vi "UI.vi"() -> ()   [LabVIEW 2017]
uses:
  <vilib>/vision/NI_Vision_Development_Module.lvlib
panel:
  out "D_damaged 4":ext
  out "D_giltch 4":ext
  out "D_damaged 3":ext
  out "D_giltch 3":ext
  out "D_damaged 2":ext
  out "D_giltch 2":ext
  out "D_damaged":ext
  out "D_giltch":ext
  in  "side length (mm)":dbl
  in  "Path":path
  in  "Main Range (Threshold)":cluster{"Lower value":sgl, "Upper value":sgl}={"Lower value"=73.0, "Upper value"=255.0}
  out "display image":T1(plugin-control)
  in  "image imshow":bool
  out "time image processing":u32
  out "time load image":u32
  out "Y Resolution":i32
  out "X Resolution":i32
  out "black image":T1(plugin-control)
  out "buffer image":T1(plugin-control)
  in  "Sub Range (Threshold)":cluster{"Lower value":sgl, "Upper value":sgl}={"Lower value"=73.0, "Upper value"=255.0}
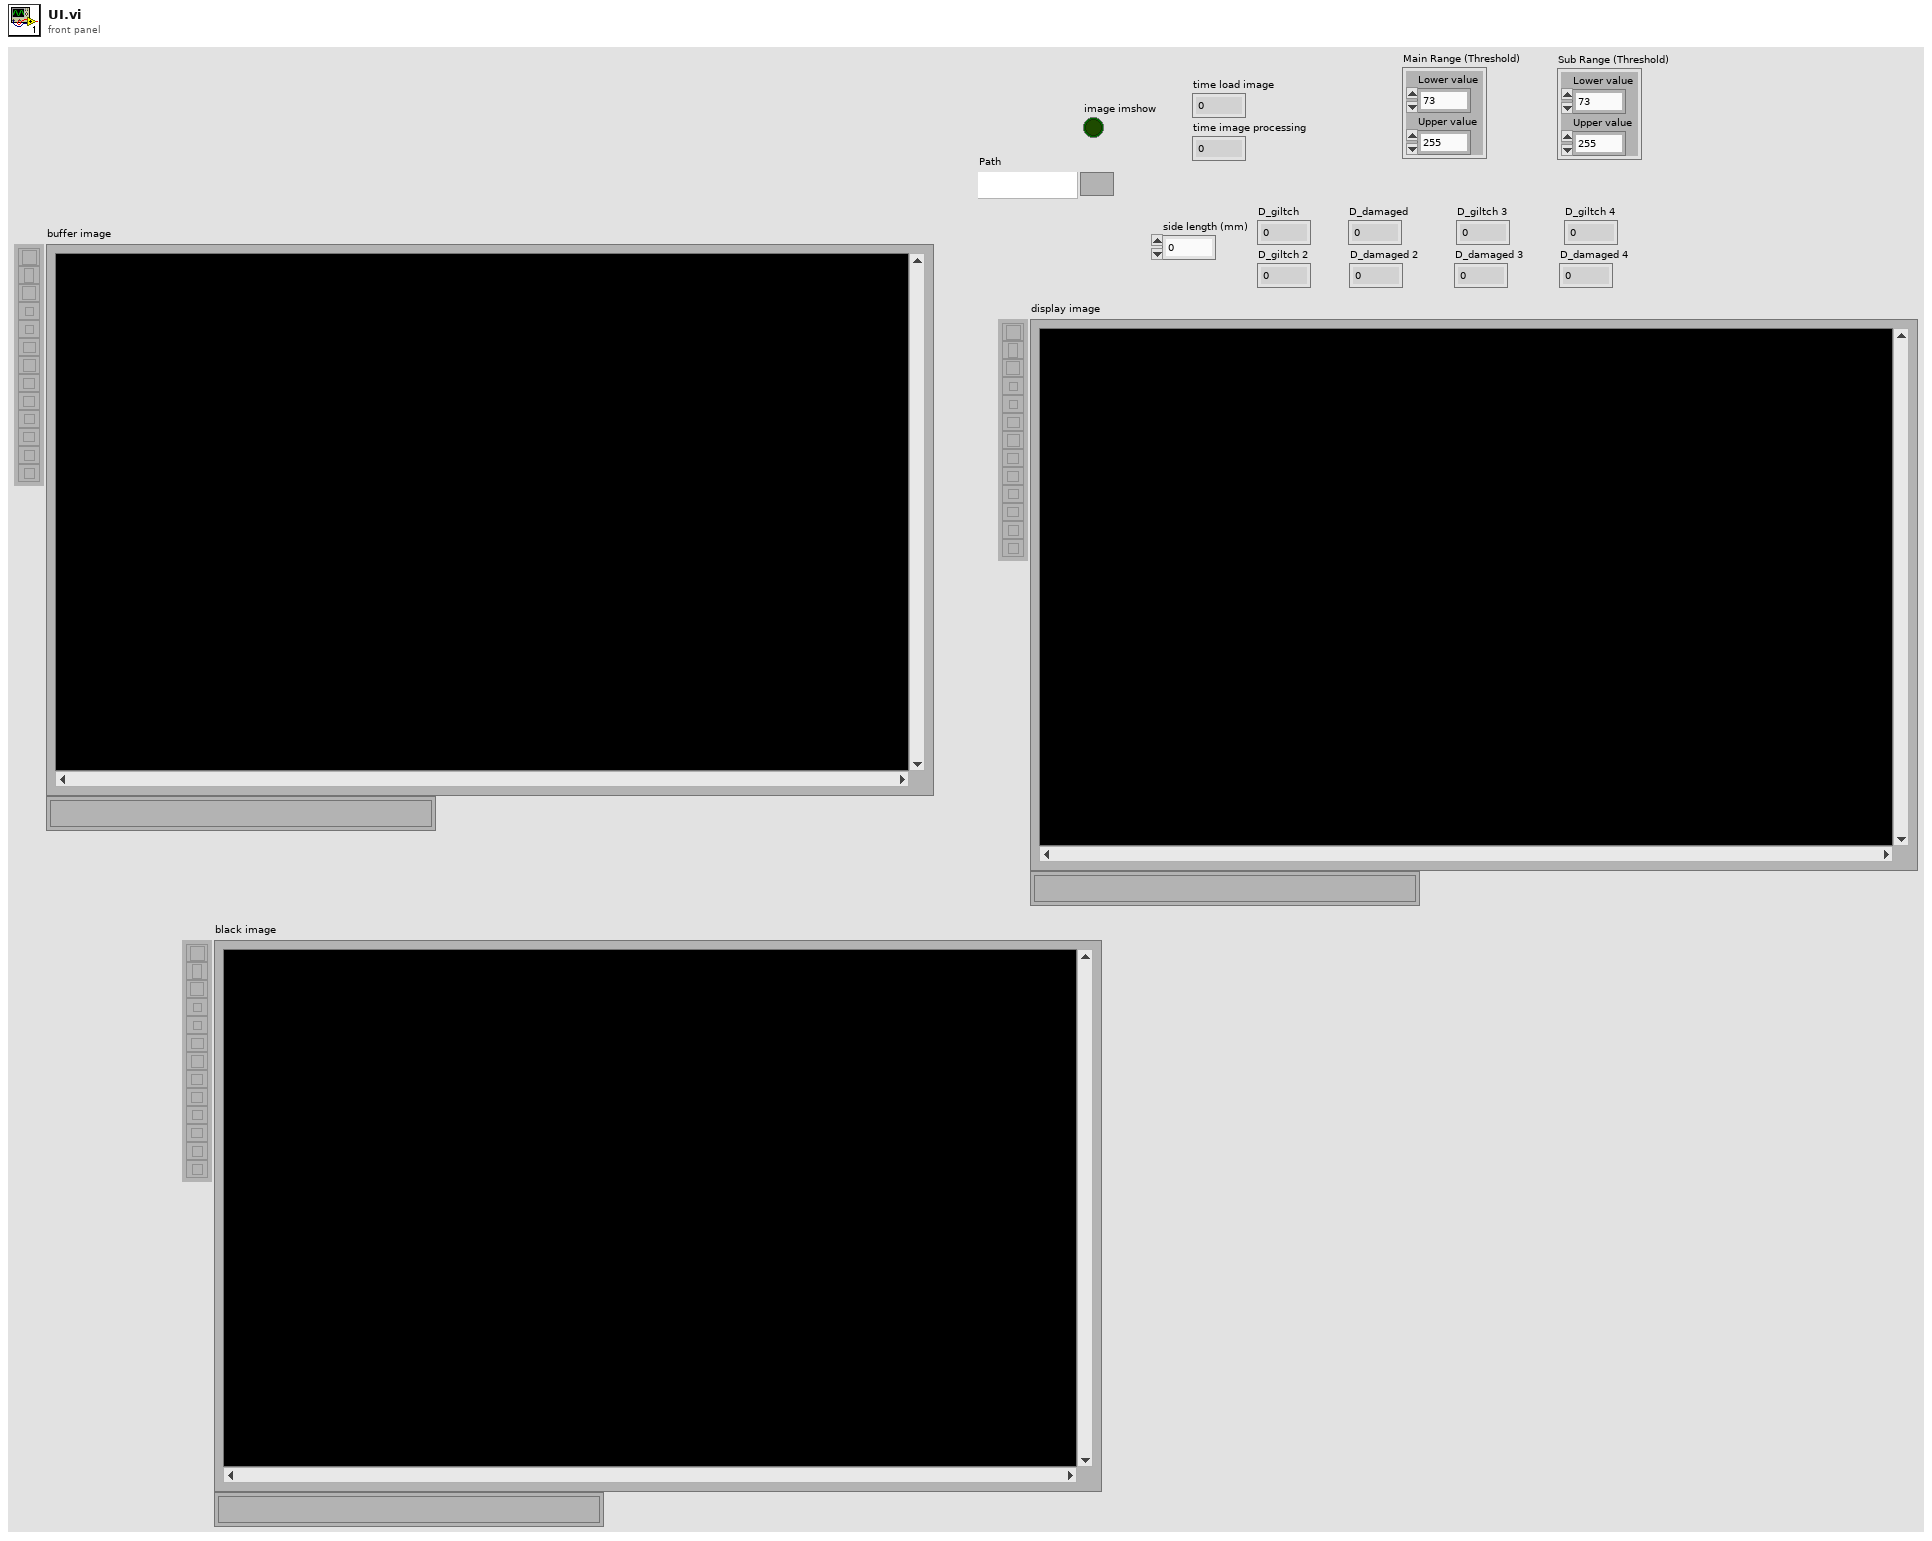
[diagram p1: front panel]
types:
  T1 = typedef "IMAQ Image.ctl" = refnum<image>
  T2 = enum32{"AutoM", "Close", "Dilate", "Erode", "Gradient", "Gradient out", "Gradient in", "Hit miss", "Open", "PClose", "POpen", "Thick", "Thin"}
  T3 = cluster{"Sigma":sgl, "HThresh":sgl, "LThres":sgl, "WindowSize":i32}
  T4 = cluster{"Number of Points":i32, "Open/Closed":i32, "Weight":dbl, "Contour Points":cluster{"X":dbl, "Y":dbl, "Curvature":dbl, "X Displacement":dbl, "Y Displacement":dbl}[]}[]
  T5 = cluster{"Left":i32, "Top":i32, "Right":i32, "Bottom":i32}
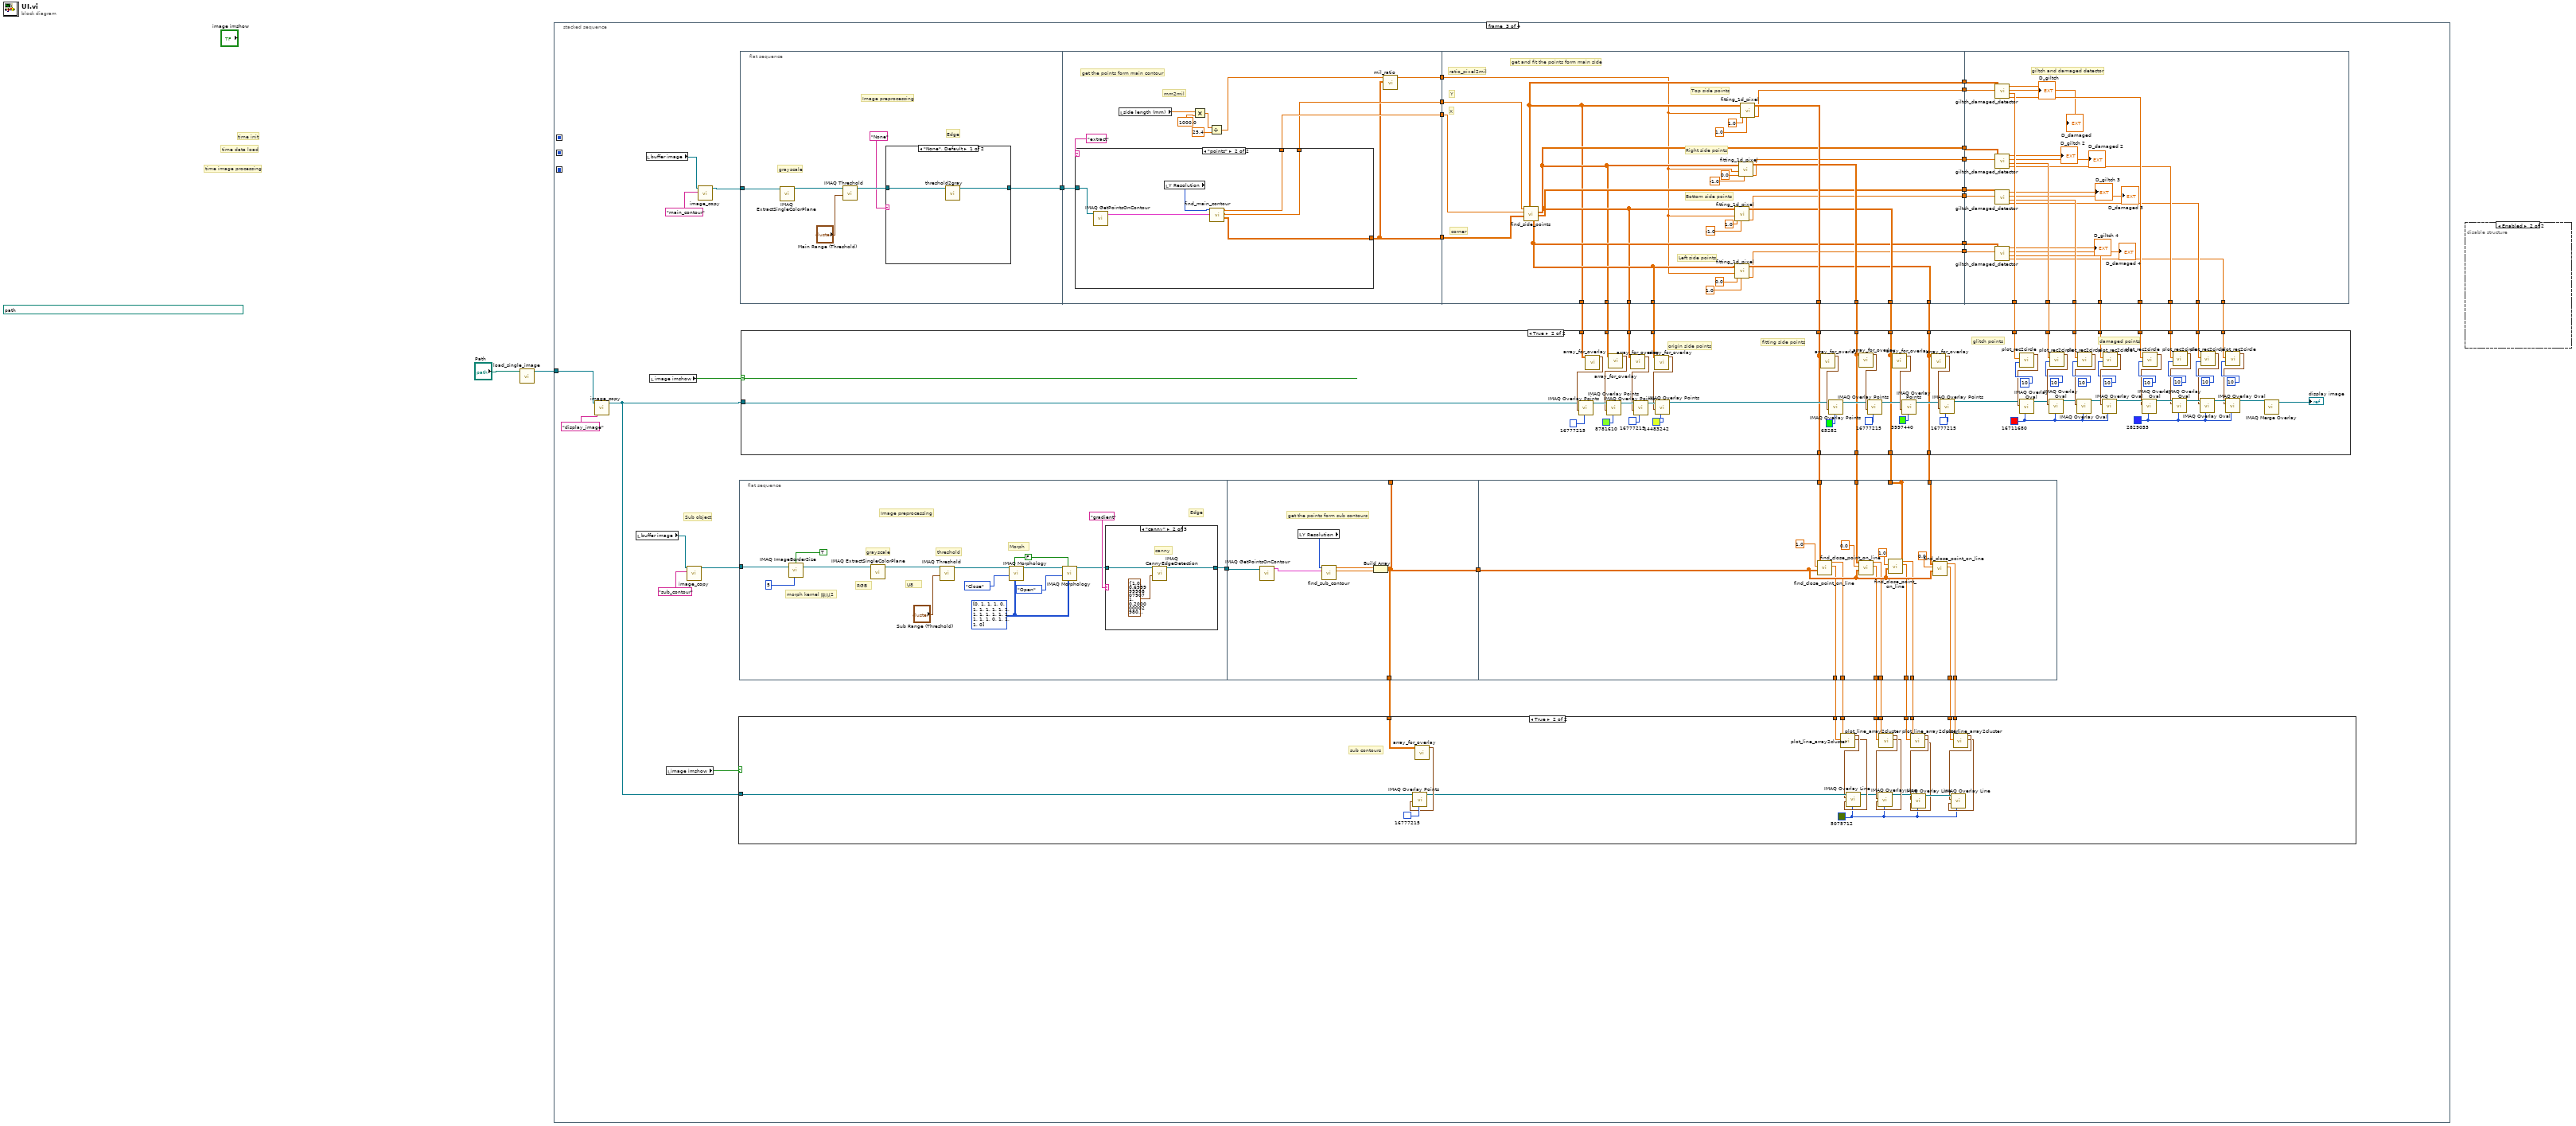
[diagram p0: block diagram]
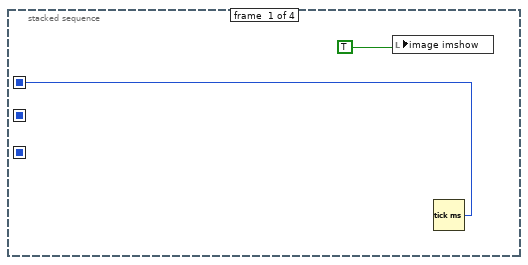
[diagram p2: hidden frame]
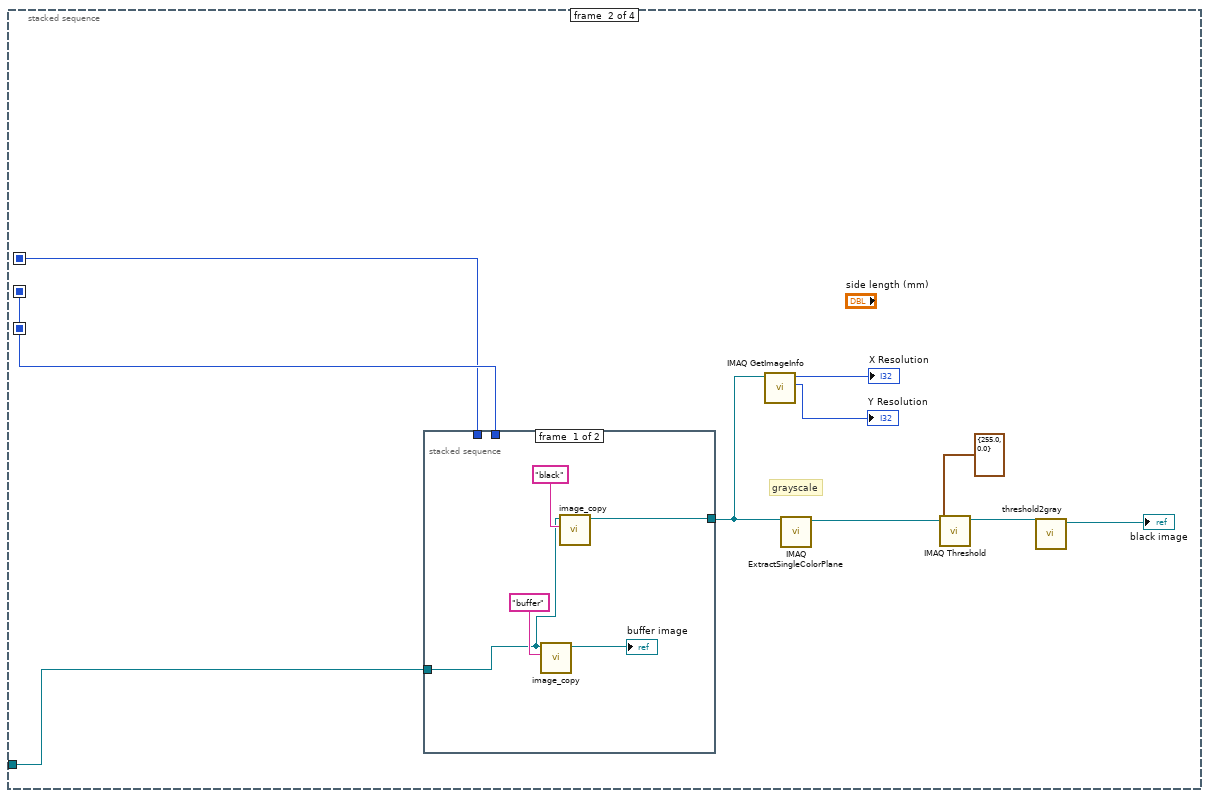
[diagram p3: hidden frame]
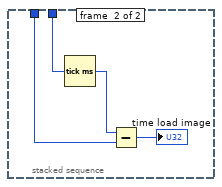
[diagram p4: hidden frame]
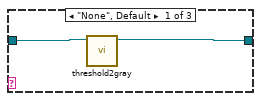
[diagram p6: hidden frame]
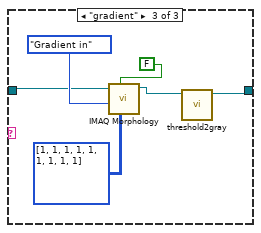
[diagram p7: hidden frame]
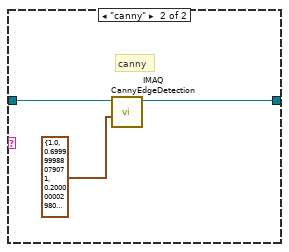
[diagram p8: hidden frame]
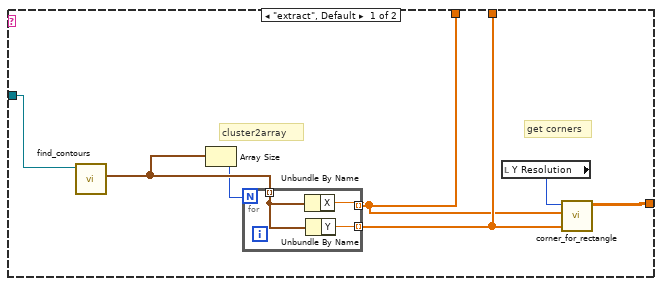
[diagram p9: hidden frame]
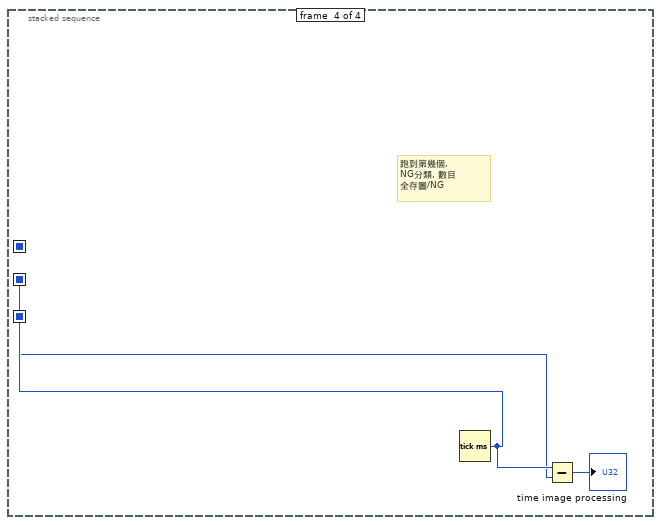
[diagram p11: hidden frame]
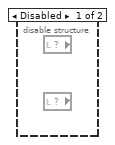
[diagram p12: hidden frame]
diagram:
  (unwired) path "X:/liteon_repeater/labview/G163良品及不良照片/labview_code/test_img/bottom-damage-1.png" ("Path")
  # "time image processing"
  # "time data load"
  # "time init"
  n1 = call "load_single_image.vi"("Path"="Path") -> ("Refnum out"=w2:T1)  [unwired: 10 in]
  n2 = stacked-sequence {
    seq-local: [w4 _ _ _] -> [_ w7 _ _]
    seq-local: [_ w8 _ _] -> [_ _ _ w311]
    seq-local: [_ _ _ w312] -> [_ _ _ _]
    tunnel: w2 -> [_ w9 w34 _]
    frame #0 {
      n3 = local write "image imshow"(TRUE) -> ()
      n4 = Tick Count (ms)() -> (millisecond timer value=w4:u32)
    }
    frame #1 {
      # "grayscale"
      n5 = stacked-sequence {
        tunnel: [w17 _] -> w12
        tunnel: w9 -> [w16 _]
        tunnel: [_ w22] -> w8
        tunnel: w7 -> [_ w21]
        frame #0 {
          n6 = call "image_copy.vi"("buffer name"="buffer" ("Image Name"), "image in"=w16) -> ("imgae out"=→"buffer image":T1)  [unwired: 9 in]
          n7 = call "image_copy.vi"("buffer name"="black" ("Image Name"), "image in"=w16) -> ("imgae out"=w17:T1)  [unwired: 9 in]
        }
        frame #1 {
          n8 = Tick Count (ms)() -> (millisecond timer value=w22:u32)
          n9 = Subtract(x=w22, y=w21) -> (x-y=→"time load image":u32)
        }
      }
      n10 = call "IMAQ GetImageInfo"("Image"=w12) -> ("Y Resolution"=→"Y Resolution":i32, "X Resolution"=→"X Resolution":i32)  [unwired: 3 in, 6 out]
      n11 = call "IMAQ ExtractSingleColorPlane"("Image Src"=w12) -> ("Image Dst Out"=w14:T1)  [unwired: 3 in, 7 out]
      n12 = call "IMAQ Threshold"("Range"=cluster{"Lower value":sgl, "Upper value":sgl} {"Lower value"=255.0, "Upper value"=0.0}, "Image Src"=w14) -> ("Image Dst Out"=w6:T1)  [unwired: 4 in, 5 out]
      n13 = call "threshold2gray.vi"("threshold image"=w6) -> ("grayscale image"=→"black image":T1)  [unwired: 10 in]
    }
    frame #2 {
      # "Sub object"
      n14 = call "image_copy.vi"("buffer name"="display_image" ("Image Name"), "image in"=w34) -> ("imgae out"=w33:T1)  [unwired: 9 in]
      n15 = local read "buffer image"() -> (w64:T1)
      n16 = local read "buffer image"() -> (w75:T1)
      n17 = local read "image imshow"() -> (w77:bool)
      n18 = local read "image imshow"() -> (w30:bool)
      n19 = call "image_copy.vi"("buffer name"="sub_contour" ("Image Name"), "image in"=w64) -> ("imgae out"=w63:T1)  [unwired: 9 in]
      n20 = call "image_copy.vi"("buffer name"="main_contour" ("Image Name"), "image in"=w75) -> ("imgae out"=w74:T1)  [unwired: 9 in]
      n21 = case shown="True" w30 {
        tunnel: w33 -> [_ w100]
        tunnel: w32 -> [_ w99]
        tunnel: w31 -> [_ w98]
        tunnel: w29 -> [_ w96]
        tunnel: w28 -> [_ w94]
        tunnel: w27 -> [_ w92]
        tunnel: w26 -> [_ w97]
        tunnel: w25 -> [_ w95]
        tunnel: w24 -> [_ w93]
        tunnel: w23 -> [_ w91]
        frame False {
        }
        frame True {
          w78 = u32 5075712 ("Color")
          # "sub contours"
          n22 = call "array_for_overlay.vi"("Array in"=w99) -> ("Array out"=w101:cluster{"X":i32, "Y":i32}[])  [unwired: 10 in]
          n23 = call "IMAQ Overlay Points"("Color"=u32 16777215, "Array of Points"=w101, "Image"=w100) -> ("Image Out"=w90:T1)  [unwired: 7 in, 1 out]
          n24 = call "plot_line_array2cluster.vi"("End Point array"=w98, "Start Point array"=w97) -> ("End Point out"=w88:cluster{"X":i32, "Y":i32}, "Start Point out"=w89:cluster{"X":i32, "Y":i32})  [unwired: 8 in]
          n25 = call "IMAQ Overlay Line"("Color"=w78, "End Point"=w88, "Start Point"=w89, "Image"=w90) -> ("Image Out"=w85:T1)  [unwired: 6 in, 1 out]
          n26 = call "plot_line_array2cluster.vi"("End Point array"=w96, "Start Point array"=w95) -> ("End Point out"=w86:cluster{"X":i32, "Y":i32}, "Start Point out"=w87:cluster{"X":i32, "Y":i32})  [unwired: 8 in]
          n27 = call "IMAQ Overlay Line"("Color"=w78, "End Point"=w86, "Start Point"=w87, "Image"=w85) -> ("Image Out"=w84:T1)  [unwired: 6 in, 1 out]
          n28 = call "plot_line_array2cluster.vi"("End Point array"=w94, "Start Point array"=w93) -> ("End Point out"=w81:cluster{"X":i32, "Y":i32}, "Start Point out"=w82:cluster{"X":i32, "Y":i32})  [unwired: 8 in]
          n29 = call "IMAQ Overlay Line"("Color"=w78, "End Point"=w81, "Start Point"=w82, "Image"=w84) -> ("Image Out"=w83:T1)  [unwired: 6 in, 1 out]
          n30 = call "plot_line_array2cluster.vi"("End Point array"=w92, "Start Point array"=w91) -> ("End Point out"=w79:cluster{"X":i32, "Y":i32}, "Start Point out"=w80:cluster{"X":i32, "Y":i32})  [unwired: 8 in]
          n31 = call "IMAQ Overlay Line"("Color"=w78, "End Point"=w79, "Start Point"=w80, "Image"=w83) -> ()  [unwired: 6 in, 2 out]
        }
      }
      n32 = flat-sequence {
        tunnel: w63 -> [w112]
        tunnel: [w108] -> w62
        tunnel: w62 -> [w134]
        tunnel: [w129] -> _
        tunnel: [w129] -> w36
        tunnel: [w129] -> w32
        tunnel: w40 -> [w145]
        tunnel: w39 -> [w149]
        tunnel: [w148] -> _
        tunnel: w38 -> [w148]
        tunnel: w37 -> [w146]
        tunnel: w36 -> [w147]
        tunnel: [w142] -> w31
        tunnel: [w141] -> w29
        tunnel: [w140] -> w28
        tunnel: [w139] -> w27
        tunnel: [w138] -> w26
        tunnel: [w137] -> w25
        tunnel: [w136] -> w24
        tunnel: [w135] -> w23
        frame #0 {
          w105 = i32[][] [[0, 1, 1, 1, 0], [1, 1, 1, 1, 1], [1, 1, 1, 1, 1], [1, 1, 1, 1, 1], [0, 1, 1, 1, 0]] ("Structuring Element")
          w106 = FALSE ("Square/Hexa (Square)")
          # "Image preprocessing"
          # "Morph"
          # "morph kernel 除以2"
          # "Edge"
          # "U8"
          # "RGB"
          # "threshold"
          # "grayscale"
          n33 = call "IMAQ ImageBorderSize"("Get/Set Status? (Set)"=TRUE, "Image"=w112, "Image border size in"=5) -> ("Image Out"=w111:T1)  [unwired: 1 in, 2 out]
          n34 = call "IMAQ ExtractSingleColorPlane"("Image Src"=w111) -> ("Image Dst Out"=w116:T1)  [unwired: 3 in, 7 out]
          n35 = call "IMAQ Threshold"("Range"="Sub Range (Threshold)", "Image Src"=w116) -> ("Image Dst Out"=w113:T1)  [unwired: 4 in, 5 out]
          n36 = call "IMAQ Morphology"("Structuring Element"=w105, "Square/Hexa (Square)"=w106, "Operation"=T2."Close", "Image Src"=w113) -> ("Image Dst Out"=w103:T1)  [unwired: 3 in, 4 out]
          n37 = call "IMAQ Morphology"("Structuring Element"=w105, "Square/Hexa (Square)"=w106, "Operation"=T2."Open", "Image Src"=w103) -> ("Image Dst Out"=w104:T1)  [unwired: 3 in, 4 out]
          n38 = case shown="\"canny\"" "gradient" {
            tunnel: [w118 w122 w123] -> w108
            tunnel: w104 -> [w119 w121 w125]
            frame "None", Default {
              n39 = call "threshold2gray.vi"("threshold image"=w119) -> ("grayscale image"=w118:T1)  [unwired: 10 in]
            }
            frame "canny" {
              # "canny"
              n40 = call "IMAQ CannyEdgeDetection"("Image Src"=w121, "Filter Parameters"=T3 {"Sigma"=1.0, "HThresh"=0.7, "LThres"=0.2, "WindowSize"=9}) -> ("Image Dst Out"=w122:T1)  [unwired: 2 in, 5 out]
            }
            frame "gradient" {
              n41 = call "IMAQ Morphology"("Structuring Element"=i32[][] [[1, 1, 1], [1, 1, 1], [1, 1, 1]], "Square/Hexa (Square)"=FALSE, "Operation"=T2."Gradient in", "Image Src"=w125) -> ("Image Dst Out"=w124:T1)  [unwired: 3 in, 4 out]
              n42 = call "threshold2gray.vi"("threshold image"=w124) -> ("grayscale image"=w123:T1)  [unwired: 10 in]
            }
          }
        }
        frame #1 {
          # "get the points form sub contours"
          n43 = call "IMAQ GetPointsOnContour"("Image (Edge Image)"=w134) -> ("Segment Information"=w133:T4)  [unwired: 3 in, 2 out]
          n44 = local read "Y Resolution"() -> (w132:i32)
          n45 = call "find_sub_contour.vi"("Segment Information"=w133, "Y Resolution"=w132) -> ("Y"=w130:dbl[], "X"=w131:dbl[])  [unwired: 8 in]
          n46 = Build Array(w131, w130) -> (w129:dbl[][])
        }
        frame #2 {
          n47 = call "find_close_point_on_line.vi"("Array in"=w147, "fitting axis"=1.0, "fitting array"=w145) -> ("XY online"=w142:dbl[], "XY point"=w138:dbl[])  [unwired: 6 in, 1 out]
          n48 = call "find_close_point_on_line.vi"("Array in"=w147, "fitting axis"=0.0, "fitting array"=w149) -> ("XY online"=w141:dbl[], "XY point"=w137:dbl[])  [unwired: 6 in, 1 out]
          n49 = call "find_close_point_on_line.vi"("Array in"=w147, "fitting axis"=1.0, "fitting array"=w148) -> ("XY online"=w140:dbl[], "XY point"=w136:dbl[])  [unwired: 6 in, 1 out]
          n50 = call "find_close_point_on_line.vi"("Array in"=w147, "fitting axis"=0.0, "fitting array"=w146) -> ("XY online"=w139:dbl[], "XY point"=w135:dbl[])  [unwired: 6 in, 1 out]
        }
      }
      n51 = flat-sequence {
        tunnel: w74 -> [w156]
        tunnel: [w153] -> w73
        tunnel: w73 -> [w172]
        tunnel: [w165] -> w72
        tunnel: [w171] -> w67
        tunnel: [w170] -> w66
        tunnel: [w163] -> w41
        tunnel: w72 -> [w213]
        tunnel: [w191] -> w71
        tunnel: [w193] -> w70
        tunnel: [w195] -> w69
        tunnel: [w197] -> w68
        tunnel: w67 -> [w212]
        tunnel: w66 -> [w211]
        tunnel: [w209] -> w61
        tunnel: [w205] -> w60
        tunnel: [w204] -> w59
        tunnel: [w203] -> w58
        tunnel: [w198] -> w57
        tunnel: [w197] -> w56
        tunnel: [w196] -> w55
        tunnel: [w195] -> w54
        tunnel: [w194] -> w53
        tunnel: [w193] -> w52
        tunnel: [w192] -> w51
        tunnel: [w191] -> w50
        tunnel: w41 -> [w190]
        tunnel: w57 -> [w237]
        tunnel: w56 -> [w236]
        tunnel: w55 -> [w235]
        tunnel: w54 -> [w234]
        tunnel: w53 -> [w233]
        tunnel: w52 -> [w232]
        tunnel: w51 -> [w231]
        tunnel: w50 -> [w230]
        tunnel: [w229] -> w49
        tunnel: [w228] -> w48
        tunnel: [w227] -> w47
        tunnel: [w226] -> w46
        tunnel: [w225] -> w45
        tunnel: [w224] -> w44
        tunnel: [w223] -> w43
        tunnel: [w222] -> w42
        frame #0 {
          # "Image preprocessing"
          # "grayscale"
          # "Edge"
          n52 = call "IMAQ ExtractSingleColorPlane"("Image Src"=w156) -> ("Image Dst Out"=w155:T1)  [unwired: 3 in, 7 out]
          n53 = call "IMAQ Threshold"("Range"="Main Range (Threshold)", "Image Src"=w155) -> ("Image Dst Out"=w154:T1)  [unwired: 4 in, 5 out]
          n54 = case shown="\"None\", Default" "None" {
            tunnel: [w158 w162] -> w153
            tunnel: w154 -> [w159 w161]
            frame "None", Default {
              n55 = call "threshold2gray.vi"("threshold image"=w159) -> ("grayscale image"=w158:T1)  [unwired: 10 in]
            }
            frame "canny" {
              # "canny"
              n56 = call "IMAQ CannyEdgeDetection"("Image Src"=w161, "Filter Parameters"=T3 {"Sigma"=1.0, "HThresh"=0.7, "LThres"=0.2, "WindowSize"=9}) -> ("Image Dst Out"=w162:T1)  [unwired: 2 in, 5 out]
            }
          }
        }
        frame #1 {
          # "mm2mil"
          # "get the points form main contour"
          n57 = case shown="\"points\"" "extract" {
            tunnel: w172 -> [w176 w189]
            tunnel: [w177 w184] -> w165
            tunnel: [w175 w185] -> w170
            tunnel: [w174 w186] -> w171
            frame "extract", Default {
              # "get corners"
              # "cluster2array"
              n58 = call "find_contours.vi"("image in"=w176) -> ("Source Image Points"=w180:cluster{"X":dbl, "Y":dbl}[])  [unwired: 9 in, 1 out]
              n59 = Array Size(array=w180) -> (size(s)=w178:i32)
              n60 = for {
                N: w178 -> [_]
                tunnel: w180 -> [w182] mode=indexing
                tunnel: [w183] -> w174 mode=indexing
                tunnel: [w181] -> w175 mode=indexing
                n61 = Unbundle By Name(w182) -> ("X"=w183:dbl)
                n62 = Unbundle By Name(w182) -> ("Y"=w181:dbl)
              }
              n63 = local read "Y Resolution"() -> (w179:i32)
              n64 = call "corner_for_rectangle.vi"("Y"=w175, "X"=w174, "Y Resolution"=w179) -> ("corner"=w177:dbl[][])  [unwired: 7 in, 1 out]
            }
            frame "points" {
              n65 = call "IMAQ GetPointsOnContour"("Image (Edge Image)"=w189) -> ("Segment Information"=w187:T4)  [unwired: 3 in, 2 out]
              n66 = local read "Y Resolution"() -> (w188:i32)
              n67 = call "find_main_contour.vi"("Segment Information"=w187, "Y Resolution"=w188) -> ("max corner"=w184:dbl[][], "Y"=w185:dbl[], "X"=w186:dbl[])  [unwired: 7 in]
            }
          }
          n68 = local read "side length (mm)"() -> (w168:dbl)
          n69 = Multiply(x=w168, y=1000.0) -> (x*y=w167:dbl)
          n70 = Divide(x=w167, y=25.4) -> (x/y=w164:dbl)
          n71 = call "mil_ratio.vi"("corner"=w165, "mil"=w164) -> ("ratio"=w163:dbl)  [unwired: 9 in]
        }
        frame #2 {
          # "corner"
          # "X"
          # "Y"
          # "ratio_pixel2mil"
          # "Left side points"
          # "Bottom side points"
          # "Right side points"
          # "Top side points"
          # "get and fit the points form main side"
          n72 = call "find_side_points.vi"("corner"=w213, "X  coords array"=w212, "Y coords array"=w211) -> ("Bottom side points"=w195:dbl[][], "Right side points"=w193:dbl[][], "Top side points"=w191:dbl[][], "Left side points"=w197:dbl[][])  [unwired: 5 in]
          n73 = call "fitting_1d_pixel.vi"("D sign"=-1.0, "fitting axis"=1.0, "ratio_pixel2mil"=w190, "array in"=w195) -> ("D"=w196:ext[], "fitting array"=w204:dbl[][])  [unwired: 6 in]
          n74 = call "fitting_1d_pixel.vi"("D sign"=1.0, "fitting axis"=0.0, "ratio_pixel2mil"=w190, "array in"=w197) -> ("D"=w198:ext[], "fitting array"=w203:dbl[][])  [unwired: 6 in]
          n75 = call "fitting_1d_pixel.vi"("D sign"=-1.0, "fitting axis"=0.0, "ratio_pixel2mil"=w190, "array in"=w193) -> ("D"=w194:ext[], "fitting array"=w205:dbl[][])  [unwired: 6 in]
          n76 = call "fitting_1d_pixel.vi"("D sign"=1.0, "fitting axis"=1.0, "ratio_pixel2mil"=w190, "array in"=w191) -> ("D"=w192:ext[], "fitting array"=w209:dbl[][])  [unwired: 6 in]
        }
        frame #3 {
          # "giltch and damaged detector"
          n77 = call "giltch_damaged_detector.vi"("D"=w231, "side points"=w230) -> ("damaged coord"=w225:dbl[], "giltch_coord"=w229:dbl[], "D_damaged"=→"D_damaged":ext, "D_giltch"=→"D_giltch":ext)  [unwired: 6 in]
          n78 = call "giltch_damaged_detector.vi"("D"=w233, "side points"=w232) -> ("damaged coord"=w224:dbl[], "giltch_coord"=w228:dbl[], "D_damaged"=→"D_damaged 2":ext, "D_giltch"=→"D_giltch 2":ext)  [unwired: 6 in]
          n79 = call "giltch_damaged_detector.vi"("D"=w235, "side points"=w234) -> ("damaged coord"=w223:dbl[], "giltch_coord"=w227:dbl[], "D_damaged"=→"D_damaged 3":ext, "D_giltch"=→"D_giltch 3":ext)  [unwired: 6 in]
          n80 = call "giltch_damaged_detector.vi"("D"=w237, "side points"=w236) -> ("damaged coord"=w222:dbl[], "giltch_coord"=w226:dbl[], "D_damaged"=→"D_damaged 4":ext, "D_giltch"=→"D_giltch 4":ext)  [unwired: 6 in]
        }
      }
      n81 = case shown="True" w77 {
        tunnel: w33 -> [_ w245]
        tunnel: w71 -> [_ w298]
        tunnel: w70 -> [_ w297]
        tunnel: w69 -> [_ w296]
        tunnel: w68 -> [_ w295]
        tunnel: w61 -> [w241 w249]
        tunnel: w60 -> [w240 w248]
        tunnel: w59 -> [w239 w247]
        tunnel: w58 -> [w238 w246]
        tunnel: w49 -> [_ w282]
        tunnel: w48 -> [_ w273]
        tunnel: w47 -> [_ w272]
        tunnel: w46 -> [_ w271]
        tunnel: w45 -> [_ w260]
        tunnel: w44 -> [_ w259]
        tunnel: w43 -> [_ w258]
        tunnel: w42 -> [_ w257]
        tunnel: [w241 w249] -> w40
        tunnel: [w240 w248] -> w39
        tunnel: [w239 w247] -> w38
        tunnel: [w238 w246] -> w37
        frame False {
        }
        frame True {
          w250 = u32 2829055 ("Color")
          w251 = u32 16711680 ("Color")
          # "damaged points"
          # "glitch points"
          # "fitting side points"
          # "origin side points"
          n82 = call "array_for_overlay.vi"("Array in"=w298) -> ("Array out"=w308:cluster{"X":i32, "Y":i32}[])  [unwired: 10 in]
          n83 = call "IMAQ Overlay Points"("Color"=u32 16777215, "Array of Points"=w308, "Image"=w245) -> ("Image Out"=w305:T1)  [unwired: 7 in, 1 out]
          n84 = call "array_for_overlay.vi"("Array in"=w297) -> ("Array out"=w301:cluster{"X":i32, "Y":i32}[])  [unwired: 10 in]
          n85 = call "IMAQ Overlay Points"("Color"=u32 8781610, "Array of Points"=w301, "Image"=w305) -> ("Image Out"=w307:T1)  [unwired: 7 in, 1 out]
          n86 = call "array_for_overlay.vi"("Array in"=w296) -> ("Array out"=w300:cluster{"X":i32, "Y":i32}[])  [unwired: 10 in]
          n87 = call "IMAQ Overlay Points"("Color"=u32 16777215, "Array of Points"=w300, "Image"=w307) -> ("Image Out"=w306:T1)  [unwired: 7 in, 1 out]
          n88 = call "array_for_overlay.vi"("Array in"=w295) -> ("Array out"=w299:cluster{"X":i32, "Y":i32}[])  [unwired: 10 in]
          n89 = call "IMAQ Overlay Points"("Color"=u32 14483242, "Array of Points"=w299, "Image"=w306) -> ("Image Out"=w283:T1)  [unwired: 7 in, 1 out]
          n90 = call "array_for_overlay.vi"("Array in"=w249) -> ("Array out"=w285:cluster{"X":i32, "Y":i32}[])  [unwired: 10 in]
          n91 = call "IMAQ Overlay Points"("Color"=u32 65282, "Array of Points"=w285, "Image"=w283) -> ("Image Out"=w288:T1)  [unwired: 7 in, 1 out]
          n92 = call "array_for_overlay.vi"("Array in"=w248) -> ("Array out"=w292:cluster{"X":i32, "Y":i32}[])  [unwired: 10 in]
          n93 = call "IMAQ Overlay Points"("Color"=u32 16777215, "Array of Points"=w292, "Image"=w288) -> ("Image Out"=w286:T1)  [unwired: 7 in, 1 out]
          n94 = call "array_for_overlay.vi"("Array in"=w247) -> ("Array out"=w293:cluster{"X":i32, "Y":i32}[])  [unwired: 10 in]
          n95 = call "IMAQ Overlay Points"("Color"=u32 3997440, "Array of Points"=w293, "Image"=w286) -> ("Image Out"=w287:T1)  [unwired: 7 in, 1 out]
          n96 = call "array_for_overlay.vi"("Array in"=w246) -> ("Array out"=w294:cluster{"X":i32, "Y":i32}[])  [unwired: 10 in]
          n97 = call "IMAQ Overlay Points"("Color"=u32 16777215, "Array of Points"=w294, "Image"=w287) -> ("Image Out"=w244:T1)  [unwired: 7 in, 1 out]
          n98 = call "plot_rec2circle.vi"("radius"=10 ("index"), "center of circle"=w282) -> ("data out"=w280:T5)  [unwired: 9 in]
          n99 = call "IMAQ Overlay Oval"("Color"=w251, "Bounding Rectangle"=w280, "Image"=w244) -> ("Image Out"=w270:T1)  [unwired: 7 in, 1 out]
          n100 = call "plot_rec2circle.vi"("radius"=10 ("index"), "center of circle"=w273) -> ("data out"=w279:T5)  [unwired: 9 in]
          n101 = call "IMAQ Overlay Oval"("Color"=w251, "Bounding Rectangle"=w279, "Image"=w270) -> ("Image Out"=w269:T1)  [unwired: 7 in, 1 out]
          n102 = call "plot_rec2circle.vi"("radius"=10 ("index"), "center of circle"=w272) -> ("data out"=w276:T5)  [unwired: 9 in]
          n103 = call "IMAQ Overlay Oval"("Color"=w251, "Bounding Rectangle"=w276, "Image"=w269) -> ("Image Out"=w268:T1)  [unwired: 7 in, 1 out]
          n104 = call "plot_rec2circle.vi"("radius"=10 ("index"), "center of circle"=w271) -> ("data out"=w275:T5)  [unwired: 9 in]
          n105 = call "IMAQ Overlay Oval"("Color"=w251, "Bounding Rectangle"=w275, "Image"=w268) -> ("Image Out"=w256:T1)  [unwired: 7 in, 1 out]
          n106 = call "plot_rec2circle.vi"("radius"=10 ("index"), "center of circle"=w260) -> ("data out"=w255:T5)  [unwired: 9 in]
          n107 = call "IMAQ Overlay Oval"("Color"=w250, "Bounding Rectangle"=w255, "Image"=w256) -> ("Image Out"=w265:T1)  [unwired: 7 in, 1 out]
          n108 = call "plot_rec2circle.vi"("radius"=10 ("index"), "center of circle"=w259) -> ("data out"=w254:T5)  [unwired: 9 in]
          n109 = call "IMAQ Overlay Oval"("Color"=w250, "Bounding Rectangle"=w254, "Image"=w265) -> ("Image Out"=w266:T1)  [unwired: 7 in, 1 out]
          n110 = call "plot_rec2circle.vi"("radius"=10 ("index"), "center of circle"=w258) -> ("data out"=w253:T5)  [unwired: 9 in]
          n111 = call "IMAQ Overlay Oval"("Color"=w250, "Bounding Rectangle"=w253, "Image"=w266) -> ("Image Out"=w267:T1)  [unwired: 7 in, 1 out]
          n112 = call "plot_rec2circle.vi"("radius"=10 ("index"), "center of circle"=w257) -> ("data out"=w252:T5)  [unwired: 9 in]
          n113 = call "IMAQ Overlay Oval"("Color"=w250, "Bounding Rectangle"=w252, "Image"=w267) -> ("Image Out"=w243:T1)  [unwired: 7 in, 1 out]
          n114 = call "IMAQ Merge Overlay"("Image Src"=w243) -> ("Image Dst Out"=→"display image":T1)  [unwired: 9 in, 1 out]
        }
      }
    }
    frame #3 {
      # "跑到第幾個, \nNG分類, 數目\n全存圖/NG"
      n115 = Tick Count (ms)() -> (millisecond timer value=w312:u32)
      n116 = Subtract(x=w312, y=w311) -> (x-y=→"time image processing":u32)
    }
  }
  n117 = disable-structure shown="Enabled" {
    frame Disabled {
      n118 = local read item#-1() -> ()  [unwired: 1 out]
      n119 = local read item#-1() -> ()  [unwired: 1 out]
    }
    frame Enabled {
    }
  }
